vi "CRYMark Frame Center.vi"() -> ()   [LabVIEW 2013]
uses:
  <vilib>/Utility/miscctls.llb/LVPositionTypeDef.ctl
  SubVI/CRYMain Sub Window Global.vi
panel:
  in  "Center":bool
  in  "sMe":string
  in  "bShow":bool=TRUE
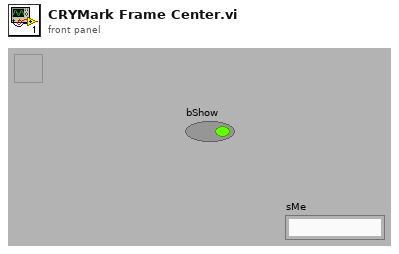
[diagram p1: front panel]
types:
  T1 = typedef "LVPositionTypeDef.ctl" = cluster{"Left":i32, "Top":i32}
  T2 = typedef "LVRectTypeDef.ctl" = cluster{"Left":i16, "Top":i16, "Right":i16, "Bottom":i16}
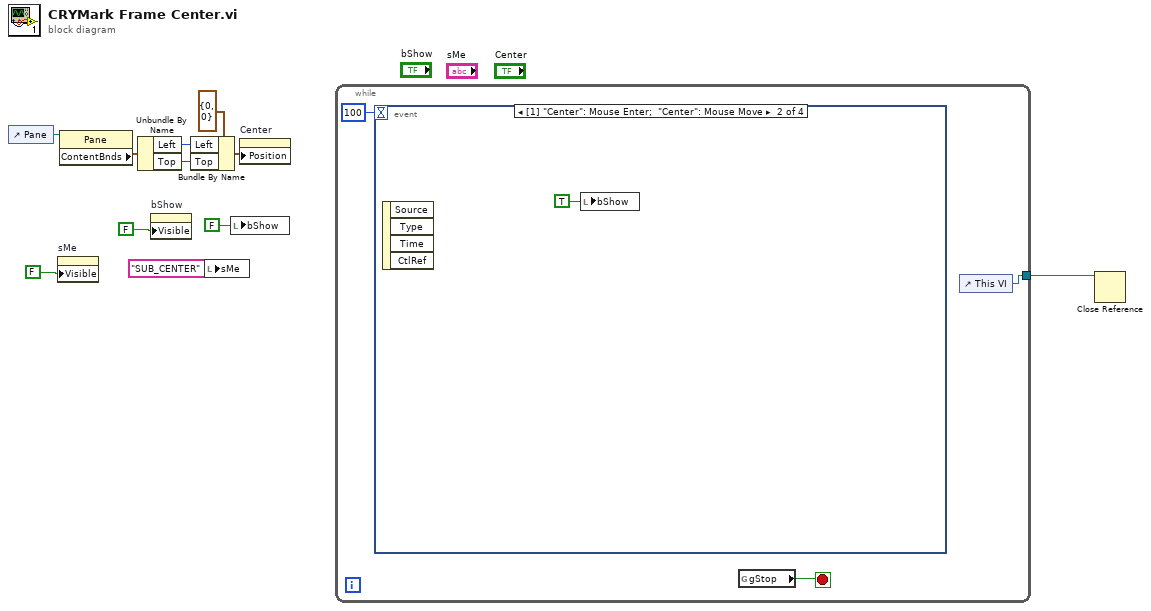
[diagram p0: block diagram]
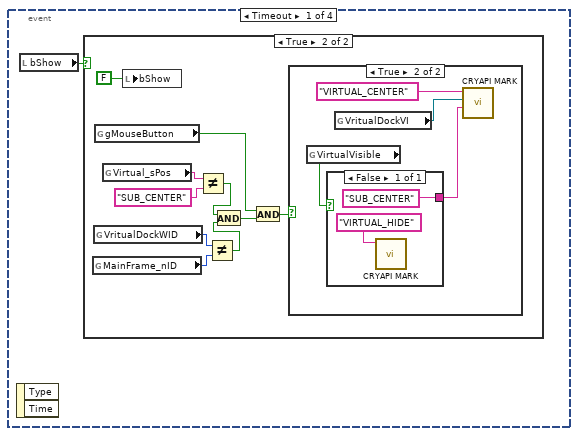
[diagram p2: hidden frame]
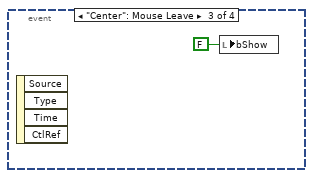
[diagram p5: hidden frame]
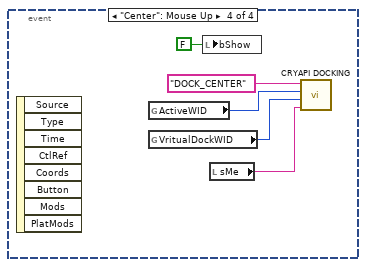
[diagram p6: hidden frame]
diagram:
  n1 = control-ref of="Pane"() -> (w11:refnum<vi>)
  n2 = property on="sMe" class="Str"("Visible"=FALSE) -> ()  [unwired: 2 in, 2 out]
  n3 = property class="Pane"(reference=w11) -> ("ContentBnds"=w10:T2)  [unwired: 1 in, 2 out]
  n4 = Unbundle By Name(w10) -> ("Left"=w9:i16, "Top"=w7:i16)
  n5 = property on="bShow" class="Bool (strict)"("Visible"=FALSE) -> ()  [unwired: 2 in, 2 out]
  n6 = Bundle By Name(cluster=T1 {"Left"=0, "Top"=0} ("Position"), "Left"=w9, "Top"=w7) -> (w2:T1)
  n7 = local write "sMe"("SUB_CENTER" ("sMe")) -> ()
  n8 = local write "bShow"(FALSE ("bShow")) -> ()
  n9 = property on="Center" class="Bool (strict)"("Position"=w2) -> ()  [unwired: 2 in, 2 out]
  n10 = while {
    tunnel: [w12] -> w1
    stop <- w13 stop-if-true
    n11 = event shown="[1] \"Center\": Mouse Enter;  \"Center\": Mouse Move" {
      selector: _ -> [_ _ _ _]
      dyn-events: _ -> [_ _ _ _]
      timeout: 100 -> [_ _ _ _]
      event Timeout {
        n12 = event-data() -> ()  [unwired: 3 out]
        n13 = local read "bShow"() -> (w15:bool)
        n14 = case shown="True" w15 {
          frame False {
          }
          frame True {
            n15 = global read "CRYMain Sub Window Global.vi" "MainFrame_nID"() -> (w23:i32)
            n16 = global read "CRYMain Sub Window Global.vi" "VritualDockWID"() -> (w22:i32)
            n17 = global read "CRYMain Sub Window Global.vi" "gMouseButton"() -> (w17:bool)
            n18 = global read "CRYMain Sub Window Global.vi" "Virtual_sPos"() -> (w21:string)
            n19 = local write "bShow"(FALSE ("bShow")) -> ()
            n20 = Not Equal?(x=w21, y="SUB_CENTER" ("sMe")) -> (x != y?=w19:bool)
            n21 = Not Equal?(x=w22, y=w23) -> (x != y?=w20:bool)
            n22 = And(x=w19, y=w20) -> (x .and. y?=w18:bool)
            n23 = And(x=w17, y=w18) -> (x .and. y?=w24:bool)
            n24 = case shown="True" w24 {
              frame False {
              }
              frame True {
                n25 = global read "CRYMain Sub Window Global.vi" "VirtualVisible"() -> (w28:bool)
                n26 = case shown="False, True" w28 {
                  tunnel: ["SUB_CENTER" ("sMe")] -> w26
                  frame False {
                    n27 = call "CRYAPI MARK.vi"("sAction"="VIRTUAL_HIDE") -> ()  [unwired: 3 in, 7 out]
                  }
                }
                n28 = global read "CRYMain Sub Window Global.vi" "VritualDockVI"() -> (w29:refnum<vi>)
                n29 = call "CRYAPI MARK.vi"("sAction"="VIRTUAL_CENTER", "mVritual_VIRef"=w29, "sData"=w26) -> ()  [unwired: 1 in, 7 out]
              }
            }
          }
        }
      }
      event "Center": Mouse Enter; "Center": Mouse Move {
        n30 = event-data() -> ()  [unwired: 5 out]
        n31 = local write "bShow"(TRUE ("bShow")) -> ()
      }
      event "Center": Mouse Leave {
        n32 = event-data() -> ()  [unwired: 5 out]
        n33 = local write "bShow"(FALSE ("bShow")) -> ()
      }
      event "Center": Mouse Up {
        n34 = event-data() -> ()  [unwired: 9 out]
        n35 = global read "CRYMain Sub Window Global.vi" "ActiveWID"() -> (w37:i32)
        n36 = global read "CRYMain Sub Window Global.vi" "VritualDockWID"() -> (w35:i32)
        n37 = local write "bShow"(FALSE ("bShow")) -> ()
        n38 = local read "sMe"() -> (w34:string)
        n39 = call "CRYAPI DOCKING.vi"("sData"=w34, "nDWinID"=w35, "nSWinID"=w37, "sAction"="DOCK_CENTER") -> ()  [unwired: 8 out]
      }
    }
    n40 = global read "CRYMain Sub Window Global.vi" "gStop"() -> (w13:bool)
    n41 = control-ref of="This VI"() -> (w12:refnum<vi>)
  }
  n42 = Close Reference(reference=w1) -> ()  [unwired: 1 in, 1 out]
